vi "Write.vi"(8 "error in (no error)":errorcluster, 10 "Modbus-Reg":u16[](array[numeric]), 11 "object in":refnum<class "Modbus-Instr.lvclass">) -> (0 "error out":errorcluster, 3 "object out":refnum<class "Modbus-Instr.lvclass">)   [LabVIEW 2021, in "Modbus-Instr.lvclass"]
doc: "Write modbus reg"
uses:
  Modbus-Instr.lvclass
  Modbus-Instr.lvclass/Modbus-Instr.ctl
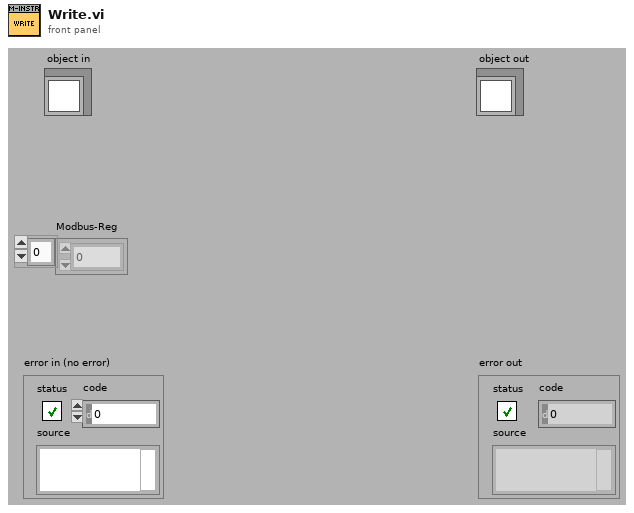
[diagram p1: front panel]
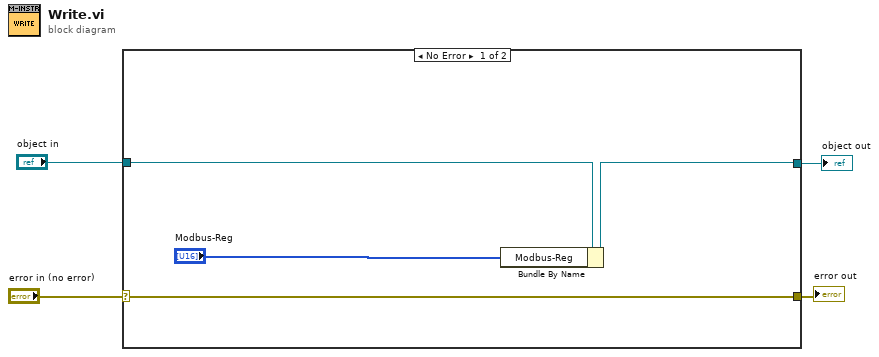
[diagram p0: block diagram]
diagram:
  n1 = case shown="No Error" "error in (no error)" {
    selector: "error in (no error)" -> [w8 w10]
    tunnel: [w8 w10] -> w3
    tunnel: [w6 w9] -> w1
    tunnel: "object in" -> [w7 w9]
    frame No Error {
      n2 = Bundle By Name(cluster=w7, "Modbus-Reg"="Modbus-Reg") -> (w6:refnum<class "Modbus-Instr.lvclass">)
    }
    frame Error {
    }
  }
  "error out" <- w3
  "object out" <- w1
